vi "User Dynamic (single).vi"(7 "User.Python.lvclass":refnum<class "User.Python.lvclass">, 8 "error in (no error)":errorcluster, 11 "XY-data":cluster{"X-array":dbl[], "Y-array":dbl[]} {"Y-array" format="%.2p"; "X-array" format="%.2p"}) -> (0 "error out":errorcluster, 3 "XY-data out":cluster{"X-array":dbl[], "Y-array":dbl[]} {"Y-array" format="%.2p"; "X-array" format="%.2p"}, 5 "User.Python.lvclass out":refnum<class "User.Python.lvclass">)   [LabVIEW 2019, in "User.Python.lvclass"]
uses:
  User.Python.lvclass
  User.Python.lvclass/User.Python.ctl
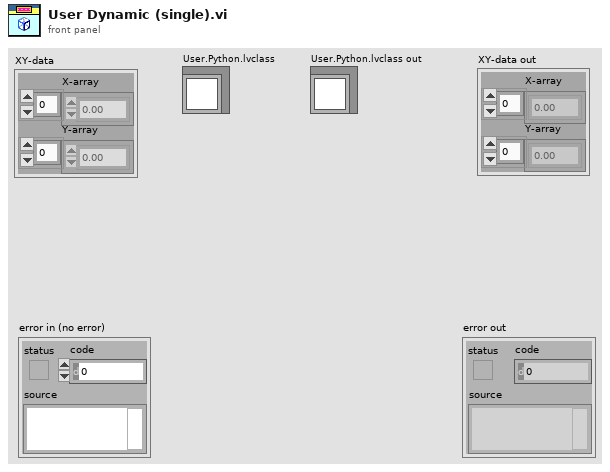
[diagram p1: front panel]
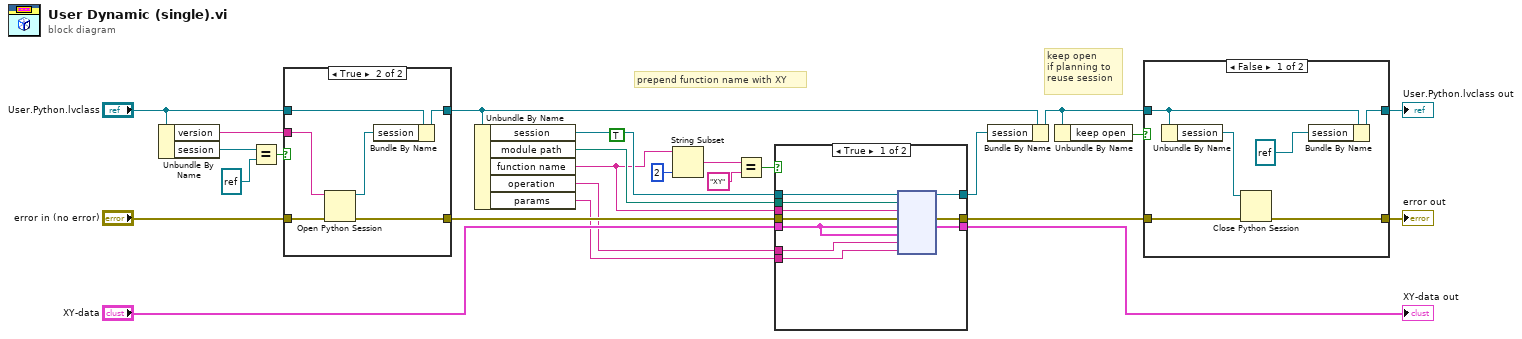
[diagram p0: block diagram]
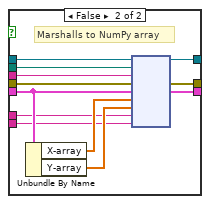
[diagram p3: hidden frame]
diagram:
  (unwired) TRUE
  # "prepend function name with XY"
  # "keep open\nif planning to \nreuse session"
  n1 = Unbundle By Name("User.Python.lvclass") -> ("version"=w19:string, "session"=w18:refnum<k35>)
  n2 = Equal?(x=w18, y=refnum<k35> refnum ("session")) -> (x = y?=w16:bool)
  n3 = case shown="True" w16 {
    tunnel: "error in (no error)" -> [w26 w33]
    tunnel: [w26 w32] -> w20
    tunnel: w19 -> [_ w31]
    tunnel: [w27 w29] -> w3
    tunnel: "User.Python.lvclass" -> [w27 w28]
    frame False {
    }
    frame True {
      n4 = Open Python Session(python version=w31, 3:w33) -> (session out=w30:refnum<k35>, error out=w32:errorcluster)  [unwired: 1 in]
      n5 = Bundle By Name(cluster=w28, "session"=w30) -> (w29:refnum<class "User.Python.lvclass">)
    }
  }
  n6 = Unbundle By Name(w3) -> ("session"=w4:refnum<k35>, "module path"=w11:path, "function name"=w2:string, "operation"=w9:string, "params"=w1:string)
  n7 = String Subset(string=w2, length (rest)=2 ("length (rest)")) -> (substring=w6:string)  [unwired: 1 in]
  n8 = Equal?(x=w6, y="XY") -> (x = y?=w5:bool)
  n9 = case shown="True" w5 {
    tunnel: [w43 w55] -> w21
    tunnel: w20 -> [w42 w54]
    tunnel: w2 -> [w41 w53]
    tunnel: w11 -> [w40 w52]
    tunnel: [w39 w51] -> w10
    tunnel: w4 -> [w38 w50]
    tunnel: w9 -> [w35 w45]
    tunnel: [w37 w49] -> w12
    tunnel: "XY-data" -> [w34 w46]
    tunnel: w1 -> [w36 w44]
    frame True {
      n10 = node(w38, w40, w41, w42, w34, w34, w35, w36) -> (w39:refnum<k35>, w43:errorcluster, w37:cluster{"X-array":dbl[], "Y-array":dbl[]})  [unwired: 3 in, 2 out]
    }
    frame False {
      # "Marshalls to NumPy array"
      n11 = Unbundle By Name(w46) -> ("X-array"=w48:dbl[], "Y-array"=w47:dbl[])
      n12 = node(w50, w52, w53, w54, w46, w48, w47, w45, w44) -> (w51:refnum<k35>, w55:errorcluster, w49:cluster{"X-array":dbl[], "Y-array":dbl[]})  [unwired: 4 in, 2 out]
    }
  }
  "XY-data out" <- w12
  n13 = Bundle By Name(cluster=w3, "session"=w10) -> (w15:refnum<class "User.Python.lvclass">)
  n14 = Unbundle By Name(w15) -> ("keep open"=w14:bool)
  n15 = case shown="False" w14 {
    tunnel: [w61 w62] -> w24
    tunnel: [w60 w63] -> w22
    tunnel: w21 -> [w59 w62]
    tunnel: w15 -> [w57 w63]
    frame False {
      n16 = Unbundle By Name(w57) -> ("session"=w58:refnum<k35>)
      n17 = Close Python Session(session in=w58, error in=w59) -> (11:w61:errorcluster)
      n18 = Bundle By Name(cluster=w57, "session"=refnum<k35> refnum) -> (w60:refnum<class "User.Python.lvclass">)
    }
    frame True {
    }
  }
  "error out" <- w24
  "User.Python.lvclass out" <- w22
